vi "publish_C4_ACS_status.vi"() -> ()   [LabVIEW 2018]
uses:
  RxTx/RxTx.lvclass
  <vilib>/addons/zeromq/socket_type.ctl
  <vilib>/addons/zeromq/zmq_socket.lvclass
  <vilib>/addons/zeromq/zmq_context.lvclass
  <vilib>/addons/zeromq/zeromq.lvlib
panel:
  out "error out":errorcluster
  out "error out 3":errorcluster
  in  "RxTx.lvclass 2":refnum<class "RxTx.lvclass">
  # "Channel 1 - ZEROMQ Communication"
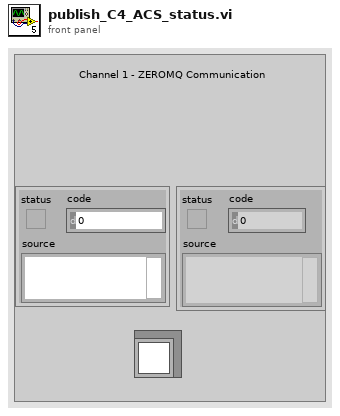
[diagram p1: front panel]
types:
  T1 = typedef "zeromq.lvlib/socket_type.ctl" = enum8{"ZMQ_PAIR", "ZMQ_PUB", "ZMQ_SUB", "ZMQ_REQ", "ZMQ_REP", "ZMQ_DEALER", "ZMQ_ROUTER", "ZMQ_PULL", "ZMQ_PUSH", "ZMQ_XPUB", "ZMQ_XSUB", "ZMQ_STREAM", "ZMQ_SERVER", "ZMQ_CLIENT", "ZMQ_RADIO", "ZMQ_DISH", "ZMQ_GATHER", "ZMQ_SCATTER", "ZMQ_DGRAM"}
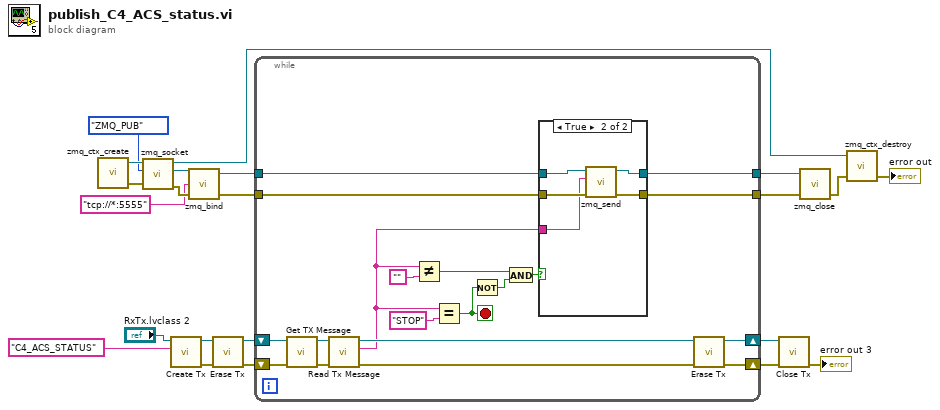
[diagram p0: block diagram]
diagram:
  n1 = call <vilib>:"zmq_ctx_create.vi"() -> ("error out"=w11:errorcluster, "context out"=w14:refnum<class "zmq_context.lvclass">)  [unwired: 4 in]
  n2 = call <vilib>:"zmq_socket.vi"("error in"=w11, "socket type"=socket_type."ZMQ_PUB", "context in"=w14) -> ("error out"=w13:errorcluster, "socket out"=w12:refnum<class "zmq_socket.lvclass">, "context out"=w5:refnum<class "zmq_context.lvclass">)  [unwired: 2 in]
  n3 = call "Create Tx.vi"("Writer Name"="C4_ACS_STATUS" ("string"), "RxTx in"="RxTx.lvclass 2") -> ("error out"=w18:errorcluster, "RxTx out"=w19:refnum<class "RxTx.lvclass">)  [unwired: 8 in]
  n4 = call <vilib>:"zmq_bind.vi"("error in"=w13, "endpoint"="tcp://*:5555", "socket in"=w12) -> ("error out"=w6:errorcluster, "socket out"=w7:refnum<class "zmq_socket.lvclass">)  [unwired: 1 in]
  n5 = call "Erase Tx.vi"("error in (no error)"=w18, "RxTx in"=w19) -> ("error out"=w15:errorcluster, "RxTx out"=w17:refnum<class "RxTx.lvclass">)  [unwired: 8 in]
  n6 = while {
    shift-right: [w41] -> w22
    shift-left: w17 -> [w35]
    shift-right: [w33] -> w16
    shift-left: w15 -> [w34]
    tunnel: w7 -> [w27]
    tunnel: w6 -> [w26]
    tunnel: [w25] -> w4
    tunnel: [w24] -> w3
    stop <- w28 stop-if-true
    n7 = call "Get TX Message.vi"("error in (no error)"=w34, "RxTx in"=w35) -> ("error out"=w40:errorcluster, "RxTx out"=w36:refnum<class "RxTx.lvclass">)  [unwired: 8 in]
    n8 = call "Read Tx Message.vi"("error in (no error)"=w40, "RxTx in"=w36) -> ("error out"=w37:errorcluster, "Tx Message"=w23:string, "RxTx out"=w38:refnum<class "RxTx.lvclass">)  [unwired: 7 in]
    n9 = Not Equal?(x=w23, y="") -> (x != y?=w31:bool)
    n10 = Equal?(x=w23, y="STOP") -> (x = y?=w28:bool)
    n11 = Not(x=w28) -> (.not. x?=w29:bool)
    n12 = And(x=w31, y=w29) -> (x .and. y?=w30:bool)
    n13 = case shown="True" w30 {
      tunnel: w27 -> [w43 w48]
      tunnel: w26 -> [w42 w47]
      tunnel: w23 -> [_ w46]
      tunnel: [w43 w45] -> w25
      tunnel: [w42 w44] -> w24
      frame False {
      }
      frame True {
        n14 = call <vilib>:"zmq_send.vi"("error in"=w47, "data"=w46, "socket in"=w48) -> ("error out"=w44:errorcluster, "socket out"=w45:refnum<class "zmq_socket.lvclass">)  [unwired: 4 in]
      }
    }
    n15 = call "Erase Tx.vi"("error in (no error)"=w37, "RxTx in"=w38) -> ("error out"=w33:errorcluster, "RxTx out"=w41:refnum<class "RxTx.lvclass">)  [unwired: 8 in]
  }
  n16 = call "Close Tx.vi"("error in (no error)"=w16, "RxTx in"=w22) -> ("error out"=→"error out 3":errorcluster)  [unwired: 8 in, 1 out]
  n17 = call <vilib>:"zmq_close.vi"("error in"=w3, "socket"=w4) -> ("error out"=w8:errorcluster)  [unwired: 3 in]
  n18 = call <vilib>:"zmq_ctx_destroy.vi"("error in"=w8, "context in"=w5) -> ("error out"=→"error out":errorcluster)  [unwired: 3 in]
